vi "PID Structure Conversion.vi"   [LabVIEW 2020, in "NI_PID_pid.lvlib"]
doc: "Converts a PID controller or controllers in Academic, Parallel, or Series form into the form (Academic) and <B>PID gains</B> units that the PID VIs expect. Wire data to the <B>proportional</B>, <B>integral</B>, or <B>derivative</B> input to determine the polymorphic instance to use, or manually select the instance."
uses:
  <vilib>/addons/control/pid/NI_PID_pid.lvlib
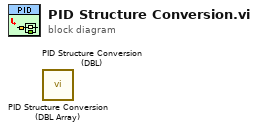
[diagram p0: block diagram]
diagram:
  n1 = call <vilib>:"PID Structure Conversion (DBL Array).vi"() -> ()  [unwired: 11 in, 1 out]
  n2 = call <vilib>:"PID Structure Conversion (DBL).vi"() -> ()  [unwired: 11 in, 1 out]
